vi "Get_niLabel.vi"(8 "error in (no error)":errorcluster, 11 "niLabel in":refnum<class "niLabel.lvclass">) -> (0 "error out":errorcluster, 2 "data":T1, 3 "niLabel out":refnum<class "niLabel.lvclass">)   [LabVIEW 2020, in "niLabel.lvclass"]
uses:
  <vilib>/AppBuilder/IB_Classes/Destination/niLabel/niLabel.lvclass
  <vilib>/AppBuilder/IB_Classes/Destination/niLabel/niLabel.lvclass/niLabel.ctl
  <vilib>/AppBuilder/IB_Classes/Destination/niLabel/IB_Dest_niLabel.ctl
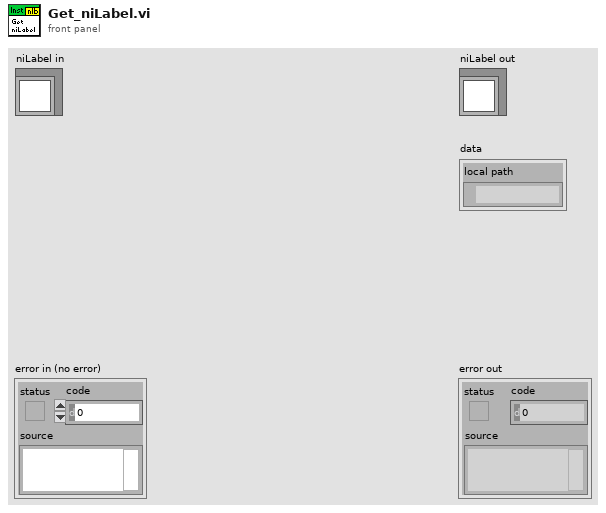
[diagram p1: front panel]
types:
  T1 = typedef "IB_Dest_niLabel.ctl" = cluster{"local path":path}
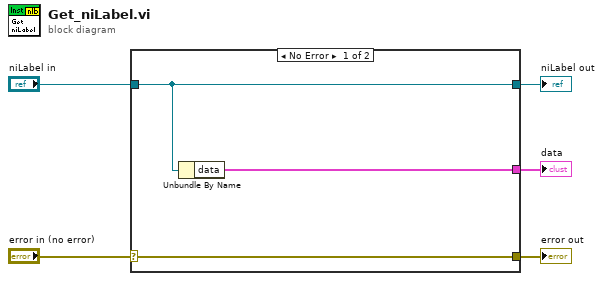
[diagram p0: block diagram]
diagram:
  n1 = case shown="No Error" "error in (no error)" {
    selector: "error in (no error)" -> [w8 w9]
    tunnel: [w8 w9] -> w4
    tunnel: [w7 w10] -> w2
    tunnel: "niLabel in" -> [w7 w10]
    tunnel: [w6 _] -> w1
    frame No Error {
      n2 = Unbundle By Name(w7) -> ("data"=w6:T1)
    }
    frame Error {
    }
  }
  "error out" <- w4
  "niLabel out" <- w2
  "data" <- w1
